vi "GIF.Read.Unpack.Interlace__ogtk.vi"(10 "Columns":i32, 11 "Interlaced":u8[](array[numeric])) -> (3 "Flat":u8[](array[numeric]))   [LabVIEW 2020]
panel:
  # "GIF.Read.Unpack.Interlace.vi\n\nRe-orders raster/rows according to GIF standard for interlaced images.\n\nPlease visit http://www.OpenG.org to learn about the\nOpen Source LabVIEW software movement.\n\nNOTICE -- YOU MUST LEAVE THIS NOTICE IN PLACE.  PER THE TERMS OF THE LICENSE BELOW, YOU MAY SUBLICENSE THIS SOFTWARE \nIN ANY WAY THAT DOES NOT CONFLICT WITH THIS LICENSE.\n\n### BSD License (http://www.opensource.org/licenses/bsd-license.php) Begin ###\n \nCopyright (c) 2007, Bill Clench <bclench@yahoo.com>\n\nAll rights reserved.\n\nRedistribution and use in source and binary forms, with or without modification, are permitted provided that the following conditions are met:\n\n    * Redistributions of source code must retain the above copyright notice, this list of conditions and the following disclaimer.\n    * Redistributions in binary form must reproduce the above copyright notice, this list of conditions and the following disclaimer in the \n       documentation and/or other materials provided with the distribution.\n    * Neither the name of SciWare, James Kring, Inc., nor the names of its contributors may be used to endorse or promote products derived \n       from this software without specific prior written permission.\n\nTHIS SOFTWARE IS PROVIDED BY THE COPYRIGHT HOLDERS AND CONTRIBUTORS \"AS IS\" AND ANY EXPRESS OR IMPLIED WARRANTIES, \nINCLUDING, BUT NOT LIMITED TO, THE IMPLIED WARRANTIES OF MERCHANTABILITY AND FITNESS FOR A PARTICULAR PURPOSE ARE \nDISCLAIMED. IN NO EVENT SHALL THE COPYRIGHT OWNER OR CONTRIBUTORS BE LIABLE FOR ANY DIRECT, INDIRECT, INCIDENTAL,\n SPECIAL, EXEMPLARY, OR CONSEQUENTIAL DAMAGES (INCLUDING, BUT NOT LIMITED TO, PROCUREMENT OF SUBSTITUTE GOODS OR \nSERVICES; LOSS OF USE, DATA, OR PROFITS; OR BUSINESS INTERRUPTION) HOWEVER CAUSED AND ON ANY THEORY OF LIABILITY, \nWHETHER IN CONTRACT, STRICT LIABILITY, OR TORT (INCLUDING NEGLIGENCE OR OTHERWISE) ARISING IN ANY WAY OUT OF THE USE \nOF THIS SOFTWARE, EVEN IF ADVISED OF THE POSSIBILITY OF SUCH DAMAGE.\n\n### BSD License End ###"
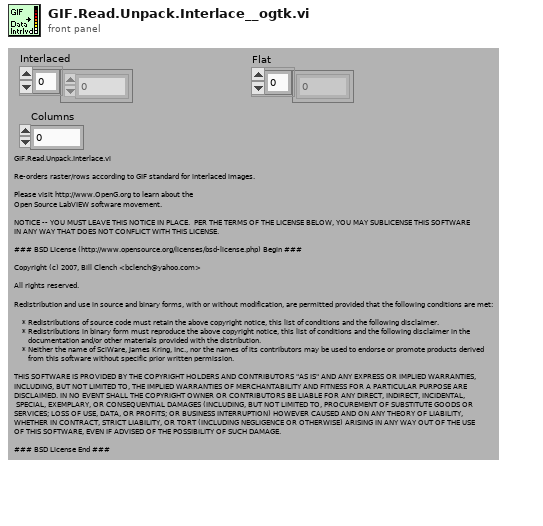
[diagram p1: front panel]
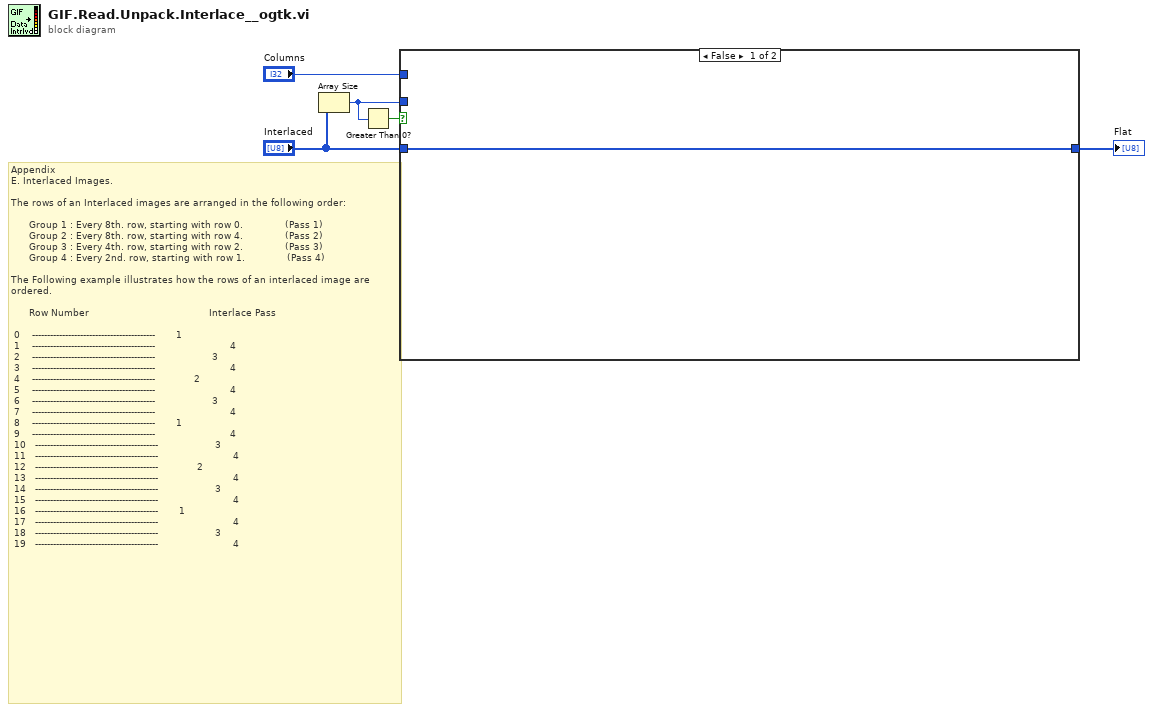
[diagram p0: block diagram]
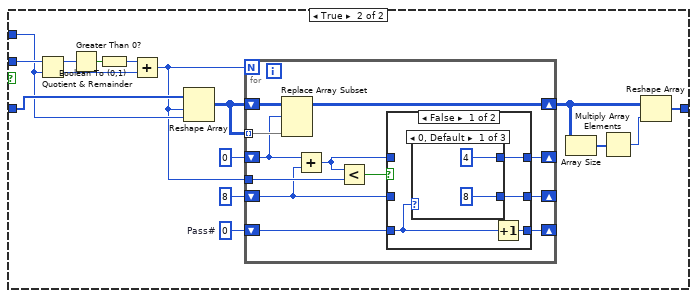
[diagram p2: hidden frame]
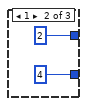
[diagram p3: hidden frame]
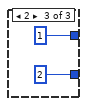
[diagram p4: hidden frame]
diagram:
  # "Appendix\nE. Interlaced Images.\n\nThe rows of an Interlaced images are arranged in the following order:\n\n      Group 1 : Every 8th. row, starting with row 0.              (Pass 1)\n      Group 2 : Every 8th. row, starting with row 4.              (Pass 2)\n      Group 3 : Every 4th. row, starting with row 2.              (Pass 3)\n      Group 4 : Every 2nd. row, starting with row 1.              (Pass 4)\n\nThe Following example illustrates how the rows of an interlaced image are\nordered.\n\n      Row Number                                        Interlace Pass\n\n 0    -----------------------------------------       1\n 1    -----------------------------------------                         4\n 2    -----------------------------------------                   3\n 3    -----------------------------------------                         4\n 4    -----------------------------------------             2\n 5    -----------------------------------------                         4\n 6    -----------------------------------------                   3\n 7    -----------------------------------------                         4\n 8    -----------------------------------------       1\n 9    -----------------------------------------                         4\n 10   -----------------------------------------                   3\n 11   -----------------------------------------                         4\n 12   -----------------------------------------             2\n 13   -----------------------------------------                         4\n 14   -----------------------------------------                   3\n 15   -----------------------------------------                         4\n 16   -----------------------------------------       1\n 17   -----------------------------------------                         4\n 18   -----------------------------------------                   3\n 19   -----------------------------------------                         4"
  n1 = Array Size(array="Interlaced") -> (size(s)=w3:i32)
  n2 = Greater Than 0?(x=w3) -> (x > 0?=w2:bool)
  n3 = case shown="False" w2 {
    tunnel: w3 -> [_ w21]
    tunnel: "Interlaced" -> [w6 w17]
    tunnel: "Columns" -> [_ w12]
    tunnel: [w6 w11] -> w1
    frame False {
    }
    frame True {
      w13 = 0  # Pass#
      n4 = Quotient & Remainder(x=w21, y=w12) -> (x-y*floor(x/y)=w22:i32, floor(x/y)=w19:i32)
      n5 = Greater Than 0?(x=w22) -> (x > 0?=w20:bool)
      n6 = Boolean To (0,1)(Boolean=w20) -> (0, 1=w18:i16)
      n7 = Add(x=w18, y=w19) -> (x+y=w7:i32)
      n8 = Reshape Array(w17, w7, w12) -> (w16:u8[][])
      n9 = for {
        N: w7 -> [_]
        shift-right: [w30] -> w10
        shift-left: w16 -> [w34]
        shift-right: [w31] -> _
        shift-left: 8 -> [w26]
        tunnel: w16 -> [w32] mode=indexing
        shift-right: [w24] -> _
        shift-left: 0 -> [w23]
        tunnel: w7 -> [w33]
        shift-right: [w28] -> _
        shift-left: w13 -> [w29]
        n10 = Replace Array Subset(array=w34, new element=w32, index (row)=w23) -> (w30:u8[][])  [unwired: 1 in]
        n11 = Add(x=w23, y=w26) -> (x+y=w25:i32)
        n12 = Less?(x=w25, y=w33) -> (x < y?=w27:bool)
        n13 = case shown="False" w27 {
          tunnel: w26 -> [_ w47]
          tunnel: w25 -> [_ w45]
          tunnel: [w36 w47] -> w31
          tunnel: [w35 w45] -> w24
          tunnel: w29 -> [w38 w46]
          tunnel: [w37 w46] -> w28
          frame False {
            n14 = case shown="0, Default" w38 {
              tunnel: [8 4 2] -> w36
              tunnel: [4 2 1] -> w35
              frame 0, Default {
              }
              frame 1 {
              }
              frame 2 {
              }
            }
            n15 = Increment(x=w38) -> (x+1=w37:i32)
          }
          frame True {
          }
        }
      }
      n16 = Array Size(array=w10) -> (size(s)=w8:i32[])
      n17 = Multiply Array Elements(1:w8) -> (0:w9:i32)
      n18 = Reshape Array(w10, w9) -> (w11:u8[])
    }
  }
  "Flat" <- w1
